vi "gcn_LVBrowser.vi"(0 "Back":bool, 1 "Forward":bool, 2 "Notice :":path, 3 "Reload":bool, 4 "Search":bool, 5 "Go":bool, 6 "SHDocVw.IWebBrowser2":refnum<k7>(container), 8 "stop":bool) -> (10 "error out":errorcluster)   [LabVIEW 2017]
doc: "To use this browser, you can type in a URL in the location field and then click on the Go button. You can also use the Back, Forward, Reload and Search buttons. This VI also has a runtime menu which is included in the library. When you run the VI, you will have File Menu and a History Menu. The file menu contains the same functionality that the buttons can do and the History menu contains a History of all the pages that you have visited in a given session.\n\nThe Invoke Node and Property Node functions are used to control the operation of the web browser. For more information on the Microsoft Web Browser Control, see Microsoft's web site (try http://support.microsoft.com/support/kb/articles/q165/2/12.asp)."
uses:
  <extravilib>/ChannelInstances/Tag-bool/Read With Abort.vi
  <extravilib>/ChannelInstances/Tag-bool/Write With Abort.vi
  <extravilib>/ChannelInstances/Tag-bool/Instantiate.vi
  <extravilib>/ChannelInstances/Tag-bool/EndpointRead.vi
  <extravilib>/ChannelInstances/Tag-bool/Endpoint.vi
  <extravilib>/ChannelInstances/Tag-bool.lvlib
panel:
  in  "Tab Control":enum32{"Browser", "Settings"}(tab)
  in  "gcn env python.exe":path=path "C:/Users/durba/.conda/envs/gcn/python.exe"
  in  "alert.py":path=path "C:/Users/durba/PycharmProjects/labview_gcn_monitor/alert.py"
  in  "run_monitor.py":path=path "C:/Users/durba/PycharmProjects/labview_gcn_monitor/run_monitor.py"
  out "standard error alert.py":string
  out "standard output alert.py":string
  out "standard output run_monitor.py":string
  out "standard error run_monitor.py":string
  out "Passing Array":string[](array[string])=["http://espn.go.com/", "http://www.natinst.com/"]
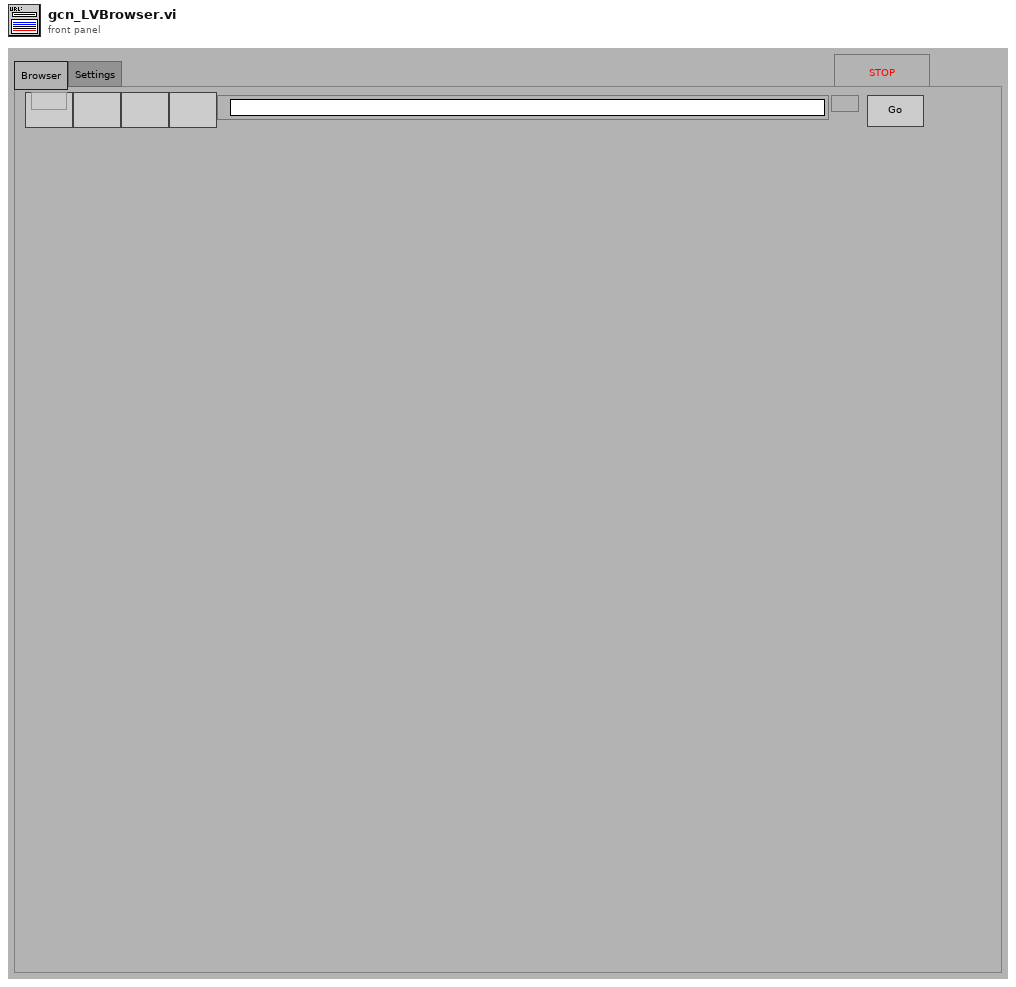
[diagram p1: front panel]
types:
  T1 = typedef "Tag-bool.lvlib/))Channel.ctl" = refnum<queue>
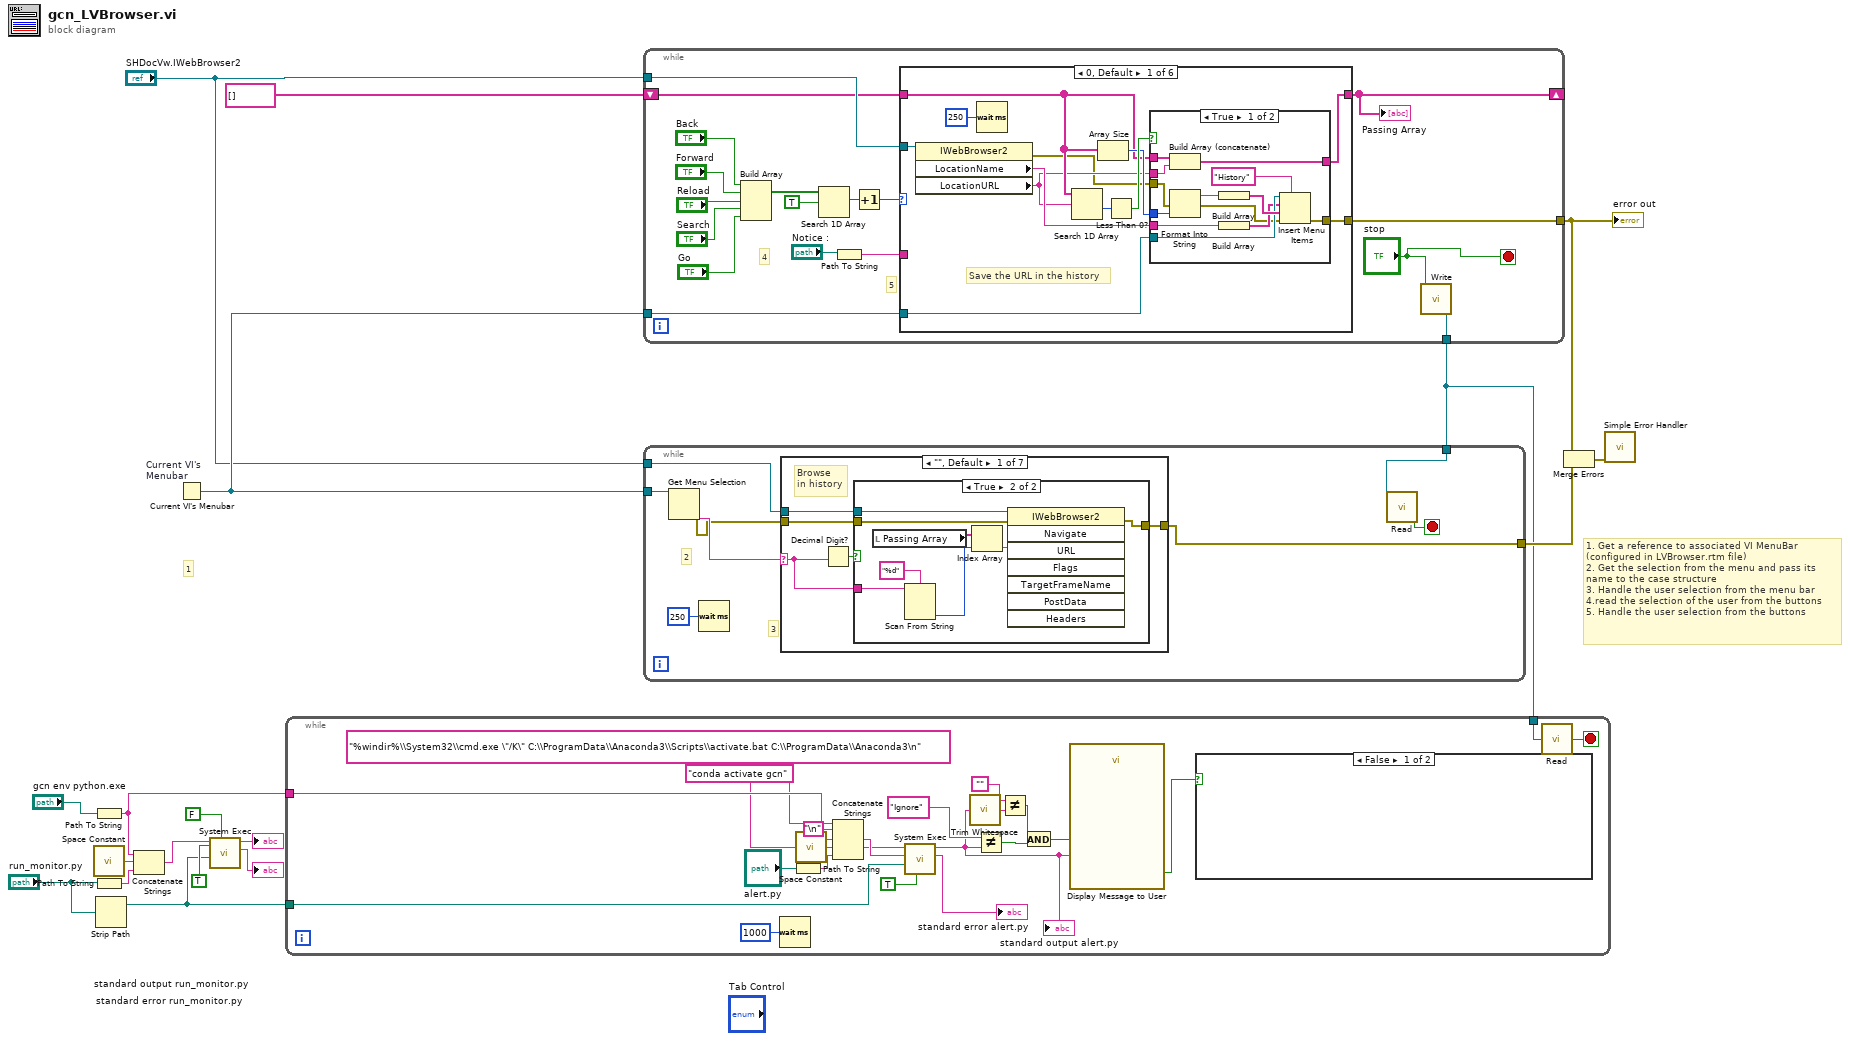
[diagram p0: block diagram]
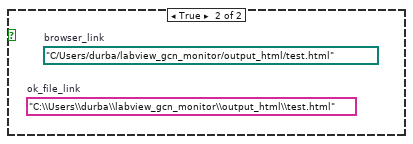
[diagram p2: hidden frame]
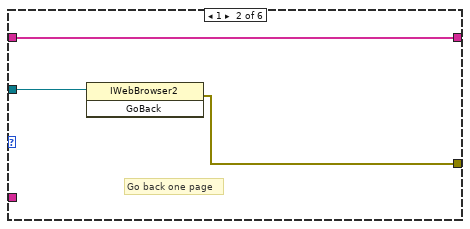
[diagram p4: hidden frame]
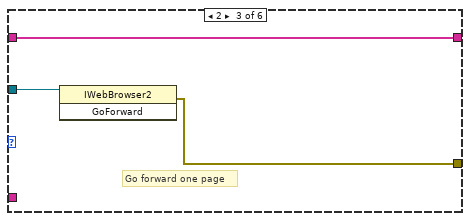
[diagram p5: hidden frame]
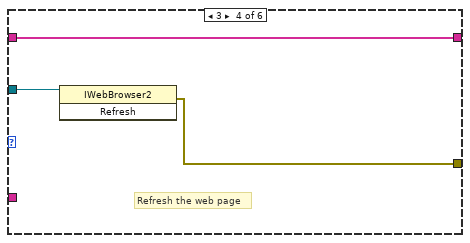
[diagram p6: hidden frame]
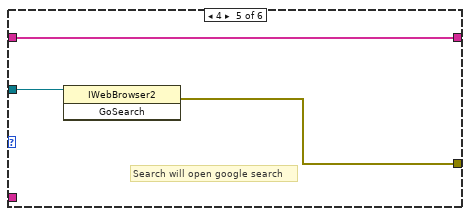
[diagram p7: hidden frame]
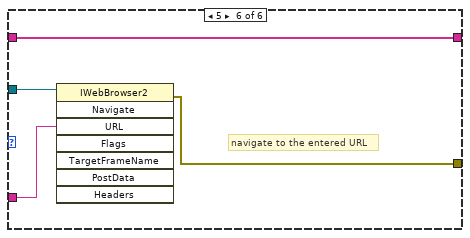
[diagram p8: hidden frame]
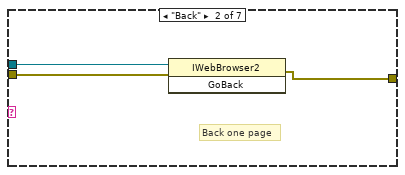
[diagram p10: hidden frame]
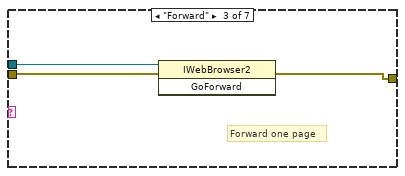
[diagram p11: hidden frame]
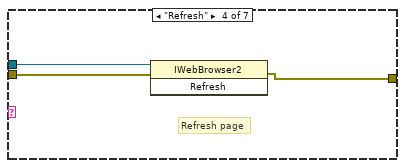
[diagram p12: hidden frame]
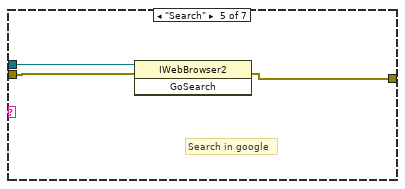
[diagram p13: hidden frame]
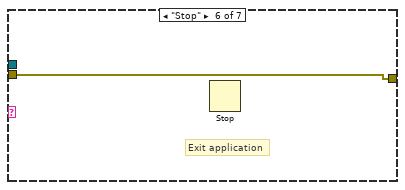
[diagram p14: hidden frame]
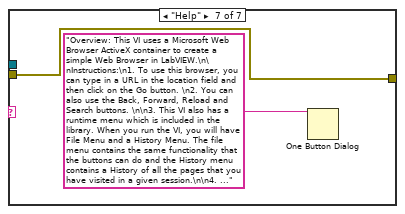
[diagram p15: hidden frame]
diagram:
  # "1. Get a reference to associated VI MenuBar \n(configured in LVBrowser.rtm file)\n2. Get the selection from the menu and pass its \nname to the case structure\n3. Handle the user selection from the menu bar\n4.read the selection of the user from the buttons\n5. Handle the user selection from the buttons"
  # "1"
  n1 = Path To String(path="gcn env python.exe") -> (string=w1:string)
  n2 = call <vilib>:"Space Constant.vi"() -> ("String"=w2:string)
  n3 = Path To String(path="run_monitor.py") -> (string=w11:string)
  n4 = Strip Path(path="run_monitor.py") -> (stripped path=w5:path)  [unwired: 1 out]
  n5 = Concatenate Strings(w1, w2, w11) -> (w9:string)
  n6 = Current VI's Menubar "Current VI's \nMenubar"() -> (w18:refnum<k9>)
  n7 = call <vilib>:"System Exec.vi"("run minimized? (F)"=TRUE, "wait until completion? (T)"=FALSE, "working directory"=w5, "command line"=w9) -> ("standard error"=→"standard error run_monitor.py":string, "standard output"=→"standard output run_monitor.py":string)  [unwired: 4 in, 2 out]
  n8 = while {
    shift-left: string[] [] -> [w25]
    shift-right: [w24] -> _
    tunnel: w18 -> [w26]
    tunnel: "SHDocVw.IWebBrowser2" -> [w27]
    tunnel: [w23] -> w15
    tunnel: [w19] -> w12
    stop <- "stop" stop-if-true
    # "5"
    # "4"
    n9 = Build Array("Back", "Forward", "Reload", "Search", "Go") -> (w31:bool[])
    n10 = Search 1D Array(1D array=w31, element=TRUE) -> (index of element=w29:i32)  [unwired: 1 in]
    n11 = Path To String(path="Notice :") -> (string=w21:string)
    n12 = Increment(x=w29) -> (x+1=w28:i32)
    n13 = case shown="0, Default" w28 {
      tunnel: w27 -> [w39 w66 w69 w71 w74 w79]
      tunnel: w26 -> [w40 _ _ _ _ _]
      tunnel: w25 -> [w44 w65 w68 w72 w75 w78]
      tunnel: [w43 w65 w68 w72 w75 w78] -> w24
      tunnel: [w38 w64 w67 w70 w73 w77] -> w23
      tunnel: w21 -> [_ _ _ _ _ w76]
      frame 0, Default {
        # "Save the URL in the history"
        n14 = property class="IWebBrowser2"(reference=w39) -> (error out=w37:errorcluster, "LocationName"=w48:string, "LocationURL"=w41:string)  [unwired: 1 in, 1 out]
        n15 = Wait (ms)(milliseconds to wait=u32 250 ("millisecond multiple")) -> ()  [unwired: 1 out]
        n16 = Search 1D Array(1D array=w44, element=w41) -> (index of element=w47:i32)  [unwired: 1 in]
        n17 = Array Size(array=w44) -> (size(s)=w45:i32)
        n18 = Less Than 0?(x=w47) -> (x < 0?=w46:bool)
        n19 = case shown="True" w46 {
          tunnel: w40 -> [w58 _]
          tunnel: w48 -> [w56 _]
          tunnel: w41 -> [w52 _]
          tunnel: w45 -> [w53 _]
          tunnel: w44 -> [w55 w63]
          tunnel: [w54 w63] -> w43
          tunnel: [w50 w62] -> w38
          tunnel: w37 -> [w49 w62]
          frame True {
            n20 = Build Array (concatenate)(w55, w52) -> (w54:string[])
            n21 = Format Into String(error in=w49, w53) -> (resulting string=w61:string, error out=w51:errorcluster)  [unwired: 2 in]
            n22 = Build Array(w61) -> (w60:string[])
            n23 = Build Array(w56) -> (w57:string[])
            n24 = Insert Menu Items(5:"History" ("menu tag"), 6:w51, 7:w60, 8:w57, 9:w58) -> (0:w50:errorcluster)  [unwired: 1 in, 2 out]
          }
          frame False {
          }
        }
      }
      frame 1 {
        # "Go back one page"
        n25 = invoke class="IWebBrowser2" method="GoBack"(reference=w66) -> (error out=w64:errorcluster)  [unwired: 2 in, 2 out]
      }
      frame 2 {
        # "Go forward one page"
        n26 = invoke class="IWebBrowser2" method="GoForward"(reference=w69) -> (error out=w67:errorcluster)  [unwired: 2 in, 2 out]
      }
      frame 3 {
        # "Refresh the web page"
        n27 = invoke class="IWebBrowser2" method="Refresh"(reference=w71) -> (error out=w70:errorcluster)  [unwired: 2 in, 2 out]
      }
      frame 4 {
        # "Search will open google search"
        n28 = invoke class="IWebBrowser2" method="GoSearch"(reference=w74) -> (error out=w73:errorcluster)  [unwired: 2 in, 2 out]
      }
      frame 5 {
        # "navigate to the entered URL"
        n29 = invoke class="IWebBrowser2" method="Navigate"(reference=w79, "URL"=w76) -> (error out=w77:errorcluster)  [unwired: 6 in, 7 out]
      }
    }
    "Passing Array" <- w24
    n30 = call <extravilib>:"Write.vi"("element"="stop") -> ("channel"=w19:T1)  [unwired: 1 out]
  }
  "error out" <- w15
  n31 = while {
    tunnel: w12 -> [w95]
    tunnel: w5 -> [w86]
    tunnel: w1 -> [w84]
    stop <- w96 stop-if-true
    n32 = Wait (ms)(milliseconds to wait=u32 1000) -> ()  [unwired: 1 out]
    n33 = Path To String(path="alert.py") -> (string=w99:string)
    n34 = call <vilib>:"Space Constant.vi"() -> ("String"=w98:string)
    n35 = Concatenate Strings("conda activate gcn" ("string"), "\n" ("string"), w84, w98, w99) -> (w83:string)
    n36 = call <vilib>:"System Exec.vi"("run minimized? (F)"=TRUE, "working directory"=w86, "standard input"=w83, "command line"="%windir%\\System32\\cmd.exe \"/K\" C:\\ProgramData\\Anaconda3\\Scripts\\activate.bat C:\\ProgramData\\Anaconda3\n") -> ("standard error"=→"standard error alert.py":string, "standard output"=w94:string)  [unwired: 4 in, 2 out]
    "standard output alert.py" <- w94
    n37 = call <vilib>:"Trim Whitespace.vi"("string"=w94) -> ("trimmed string"=w89:string)  [unwired: 1 in]
    n38 = Not Equal?(x="Ignore", y=w94) -> (x != y?=w91:bool)
    n39 = Not Equal?(x="", y=w89) -> (x != y?=w92:bool)
    n40 = And(x=w92, y=w91) -> (x .and. y?=w90:bool)
    n41 = call "Display Message to User"("Enable"=w90, "Message"=w94) -> ("OK"=w101:bool)  [unwired: 8 in, 1 out]
    n42 = case shown="False" w101 {
      frame False {
      }
      frame True {
        (unwired) path "C:/Users/durba/labview_gcn_monitor/output_html/test.html"  # browser_link
        (unwired) "C:\\Users\\durba\\labview_gcn_monitor\\output_html\\test.html"  # ok_file_link
      }
    }
    n43 = call <extravilib>:"Read.vi"("channel"=w95) -> ("element"=w96:bool)  [unwired: 1 in, 1 out]
  }
  n44 = while {
    tunnel: w18 -> [w109]
    tunnel: "SHDocVw.IWebBrowser2" -> [w107]
    tunnel: [w104] -> w14
    tunnel: w12 -> [w103]
    stop <- w102 stop-if-true
    # "3"
    # "2"
    n45 = Get Menu Selection(0:w109) -> (6:w108:string, 8:w105:errorcluster)  [unwired: 3 in, 3 out]
    n46 = Wait (ms)(milliseconds to wait=u32 250 ("millisecond multiple")) -> ()  [unwired: 1 out]
    n47 = case shown="\"\", Default" w108 {
      selector: w108 -> [w112 _ _ _ _ _ _]
      tunnel: w107 -> [w114 w126 w129 w132 w135 _ _]
      tunnel: w105 -> [w111 w125 w128 w131 w134 w136 w137]
      tunnel: [w110 w124 w127 w130 w133 w136 w137] -> w104
      frame "", Default {
        # "Browse\nin history"
        n48 = Decimal Digit?(1:w112) -> (0:w113:bool)
        n49 = case shown="True" w113 {
          tunnel: w114 -> [_ w123]
          tunnel: w112 -> [_ w119]
          tunnel: w111 -> [w115 w117]
          tunnel: [w115 w116] -> w110
          frame False {
          }
          frame True {
            n50 = local read "Passing Array"() -> (w122:string[])
            n51 = Scan From String(format string="%d", input string=w119) -> (output 1=w118:i32)  [unwired: 3 in, 3 out]
            n52 = Index Array(array=w122, index=w118) -> (element=w121:string)
            n53 = invoke class="IWebBrowser2" method="Navigate"(reference=w123, error in=w117, "URL"=w121) -> (error out=w116:errorcluster)  [unwired: 5 in, 7 out]
          }
        }
      }
      frame "Back" {
        # "Back one page"
        n54 = invoke class="IWebBrowser2" method="GoBack"(reference=w126, error in=w125) -> (error out=w124:errorcluster)  [unwired: 1 in, 2 out]
      }
      frame "Forward" {
        # "Forward one page"
        n55 = invoke class="IWebBrowser2" method="GoForward"(reference=w129, error in=w128) -> (error out=w127:errorcluster)  [unwired: 1 in, 2 out]
      }
      frame "Refresh" {
        # "Refresh page"
        n56 = invoke class="IWebBrowser2" method="Refresh"(reference=w132, error in=w131) -> (error out=w130:errorcluster)  [unwired: 1 in, 2 out]
      }
      frame "Search" {
        # "Search in google"
        n57 = invoke class="IWebBrowser2" method="GoSearch"(reference=w135, error in=w134) -> (error out=w133:errorcluster)  [unwired: 1 in, 2 out]
      }
      frame "Stop" {
        # "Exit application"
        n58 = Stop() -> ()  [unwired: 1 in]
      }
      frame "Help" {
        n59 = One Button Dialog(message="Overview: This VI uses a Microsoft Web Browser ActiveX container to create a simple Web Browser in LabVIEW.\n\nInstructions:\n1. To use this browser, you can type in a URL in the location field and then click on the Go button. \n2. You can also use the Back, Forward, Reload and Search buttons. \n\n3. This VI also has a runtime menu which is included in the library. When you run the VI, you will have File Menu and a History Menu. The file menu contains the same functionality that the buttons can do and the History menu contains a History of all the pages that you have visited in a given session.\n\n4. To Stop Execution, Click on File>> Stop") -> ()  [unwired: 1 in, 1 out]
      }
    }
    n60 = call <extravilib>:"Read.vi"("channel"=w103) -> ("element"=w102:bool)  [unwired: 1 in, 1 out]
  }
  n61 = Merge Errors(w15, w14) -> (w13:errorcluster)
  n62 = call <vilib>:"Simple Error Handler.vi"("error in (no error)"=w13) -> ()  [unwired: 4 in, 5 out]
